vi "Get Power Supply Specifications.vi"(8 "error in (no error)":errorcluster, 11 "N5745A in":refnum<class "5745A.lvclass">) -> (0 "error out":errorcluster, 2 "Limits and Protections":T1 {"Voltage Limit" format="%.3f"; "UVL" format="%.3f"; "OVP" format="%.3f"; "Current Limit" format="%.3f"}, 3 "N5745A out":refnum<class "5745A.lvclass">)   [LabVIEW 2018, in "5745A.lvlib" / "5745A.lvclass"]
doc: "This method gets the instrument's Model, Max. Voltage rating, Max.Current rating, Limits and Protection settings."
uses:
  5745A.lvclass
  Custom Controls/Limits and Protections.ctl
  5745A.lvclass/5745A.ctl
  builds/Power_Supply.lvlibp/Power Supply.lvclass
  C:/Users/Ron.Dexter.LUMINARTECH/Desktop/builds/Power_Supply.lvlibp/Power Supply.lvclass
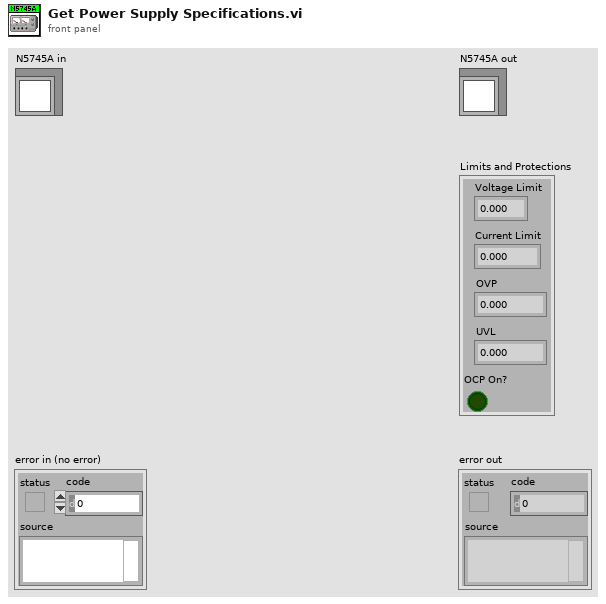
[diagram p1: front panel]
types:
  T1 = typedef "5745A.lvlib/5745A.lvclass/Limits and Protections.ctl" = cluster{"OCP On?":bool, "Current Limit":dbl, "OVP":dbl, "UVL":dbl, "Voltage Limit":dbl}
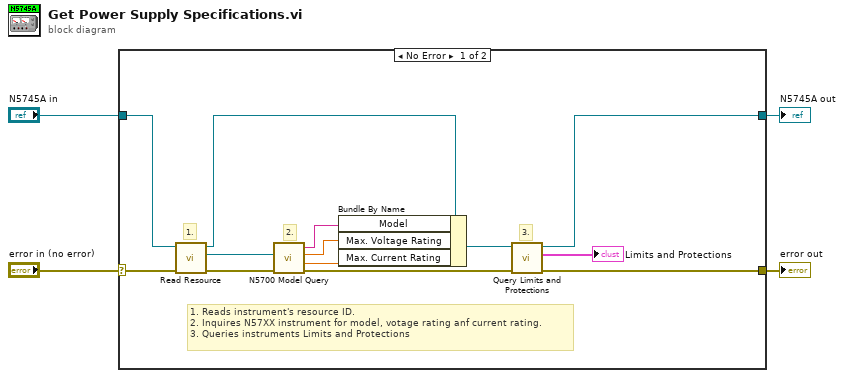
[diagram p0: block diagram]
diagram:
  n1 = case shown="No Error" "error in (no error)" {
    selector: "error in (no error)" -> [w17 w19]
    tunnel: [w8 w19] -> w3
    tunnel: [w6 w18] -> w1
    tunnel: "N5745A in" -> [w16 w18]
    frame No Error {
      # "3."
      # "1. Reads instrument's resource ID.\n2. Inquires N57XX instrument for model, votage rating anf current rating.\n3. Queries instruments Limits and Protections"
      # "2."
      # "1."
      n2 = call "Read Resource.vi"("error in"=w17, "Power Supply in"=w16) -> ("error out"=w14:errorcluster, "Resource"=w15:refnum<visa-resource-name>, "Power Supply out"=w10:refnum<class "5745A.lvclass">)  [unwired: 7 in]
      n3 = call <instrlib>:"N5700 Model Query.vi"("error"=w14, "VISA"=w15) -> ("error out"=w9:errorcluster, "Current Rating"=w13:dbl, "Voltage Rating"=w12:dbl, "Model"=w11:string)  [unwired: 2 in, 1 out]
      n4 = Bundle By Name(cluster=w10, "Model"=w11, "Max. Voltage Rating"=w12, "Max. Current Rating"=w13) -> (w7:refnum<class "5745A.lvclass">)
      n5 = call "Query Limits and Protections.vi"("error in (no error)"=w9, "N5745A in"=w7) -> ("error out"=w8:errorcluster, "Limits and Protections"=→"Limits and Protections":T1, "N5745A out"=w6:refnum<class "5745A.lvclass">)  [unwired: 7 in]
    }
    frame Error {
    }
  }
  "error out" <- w3
  "N5745A out" <- w1
